vi "Get DQMH  Item Tag.vi"(8 "error in":errorcluster, 11 "Path":path) -> (0 "error out":errorcluster, 3 "DQMH Tag":string)   [LabVIEW 2020, in "Panther Dashboard.lvlib"]
uses:
  Panther Dashboard.lvlib
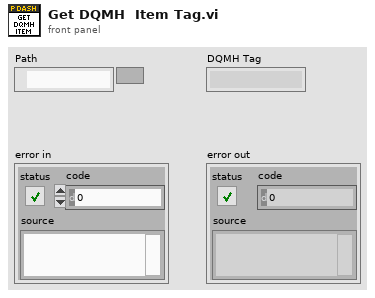
[diagram p1: front panel]
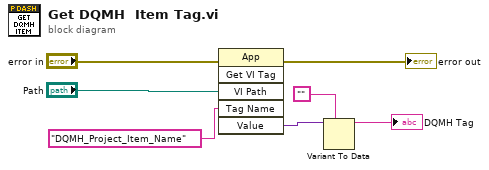
[diagram p0: block diagram]
diagram:
  n1 = invoke class="App" method="Get VI Tag"(error in="error in", "VI Path"="Path", "Tag Name"="DQMH_Project_Item_Name") -> (error out=→"error out":errorcluster, "Value"=w4:variant)  [unwired: 3 in, 4 out]
  n2 = Variant To Data(type="", Variant=w4) -> (data=→"DQMH Tag":string)  [unwired: 1 in, 1 out]
